vi "QR Code_Read QR Code Setting.vi"(8 "error in":errorcluster, 11 "Buffer Data In":T9) -> (0 "error out":errorcluster, 2 "QR Code Setting":T1={"QR Search Options"={"Rotation Mode"=enum."Unlimited", "Skip Location?"=FALSE, "Edge Threshold"=30, "Demodulation Mode"=-2, "Cell Sample Size"=-2, "Cell Filter Mode"=-2, "Skew Degrees Allowed"=5}, "QR Description Options"={"Matrix Size (cells)"=0, "Barcode Polarity"=-2, "Mirror Mode"=-2, "QR Model"=0}, "QR Code Cell Size (pixels)"={"Minimum Size"=3, "Maximum Size"=7}} {"QR Description Options"."Mirror Mode" items=["Auto-detect"=-2, "Normal"=0, "Mirrored"=1]; "QR Description Options"."Matrix Size (cells)" items=["Auto-detect"=0, "11x11 - Version 1 (Micro QR Only)"=11, "13x13 - Version 2 (Micro QR Only)"=13, "15x15 - Version 3 (Micro QR Only)"=15, "17x17 - Version 4 (Micro QR Only)"=17, "21x21 - Version 1"=21, "25x25 - Version 2"=25, "29x29 - Version 3"=29, "33x33 - Version 4"=33, "37x37 - Version 5"=37, "41x41 - Version 6"=41, "45x45 - Version 7"=45, "49x49 - Version 8"=49, "53x53 - Version 9"=53, "57x57 - Version 10"=57, "61x61 - Version 11"=61, "65x65 - Version 12"=65, "69x69 - Version 13"=69, "73x73 - Version 14"=73, "77x77 - Version 15"=77, "81x81 - Version 16"=81, "85x85 - Version 17"=85, "89x89 - Version 18"=89, "93x93 - Version 19"=93, "97x97 - Version 20"=97, "101x101 - Version 21"=101, "105x105 - Version 22"=105, "109x109 - Version 23"=109, "113x113 - Version 24"=113, "117x117 - Version 25"=117, "121x121 - Version 26"=121, "125x125 - Version 27"=125, "129x129 - Version 28"=129, "133x133 - Version 29"=133, "137x137 - Version 30"=137, "141x141 - Version 31"=141, "145x145 - Version 32"=145, "149x149 - Version 33"=149, "153x153 - Version 34"=153, "157x157 - Version 35"=157, "161x161 - Version 36"=161, "165x165 - Version 37"=165, "169x169 -  Version 38"=169, "173x173 - Version 39"=173, "177x177 - Version 40"=177]; "QR Description Options"."QR Model" items=["Auto-detect", "Micro", "Model 1", "Model 2"]; "QR Description Options"."Barcode Polarity" items=["Auto-detect"=-2, "Black on White"=0, "White on Black"=1]; "QR Search Options"."Cell Filter Mode" items=["Auto-detect"=-2, "Average"=0, "Median"=1, "Central Average"=2, "High Average"=3, "Low Average"=4, "Very High Average"=5, "Very Low Average"=6, "All Filters"=8]; "QR Search Options"."Cell Sample Size" items=["Auto-detect"=-2, "1x1"=1, "2x2"=2, "3x3"=3, "4x4"=4, "5x5"=5, "6x6"=6, "7x7"=7]; "QR Search Options"."Demodulation Mode" items=["Auto-detect"=-2, "Histogram"=0, "Local Contrast"=1, "Combination"=2, "All"=3]}, 3 "Buffer Data Out":T9)   [LabVIEW 2016]
uses:
  Data Def/QR Code_Buffer Data.ctl
  <vilib>/vision/Image Controls.llb/IMAQ Image.ctl
  Data Def/QR Code_QR Code Setting.ctl
  <vilib>/vision/Instrument.llb/QR Code Search Options.ctl
  <vilib>/vision/Instrument.llb/Demodulation Mode.ctl
  <vilib>/vision/Instrument.llb/Cell Sample Size.ctl
  <vilib>/vision/Instrument.llb/Cell Filter Mode.ctl
  <vilib>/vision/Instrument.llb/QR Code Description Options.ctl
  <vilib>/vision/Instrument.llb/Data Matrix Polarity.ctl
  <vilib>/vision/Instrument.llb/QR Code Model Type.ctl
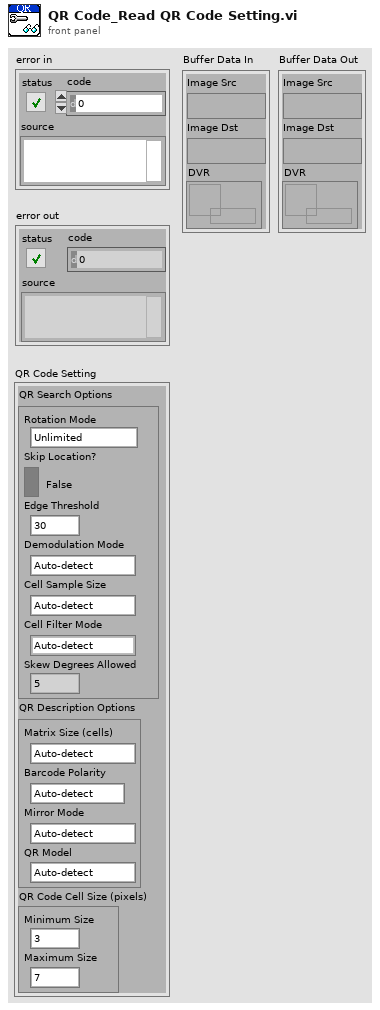
[diagram p1: front panel]
types:
  T1 = typedef "QR Code_QR Code Setting.ctl" = cluster{"QR Search Options":T2, "QR Description Options":T6, "QR Code Cell Size (pixels)":cluster{"Minimum Size":u32, "Maximum Size":u32}}
  T2 = typedef "QR Code Search Options.ctl" = cluster{"Rotation Mode":enum32{"Unlimited", "0 Degrees", "90 Degrees", "180 Degrees", "270 Degrees"}, "Skip Location?":bool, "Edge Threshold":u32, "Demodulation Mode":T3, "Cell Sample Size":T4, "Cell Filter Mode":T5, "Skew Degrees Allowed":u32}
  T3 = typedef "Demodulation Mode.ctl" = i32
  T4 = typedef "Cell Sample Size.ctl" = i32
  T5 = typedef "Cell Filter Mode.ctl" = i32
  T6 = typedef "QR Code Description Options.ctl" = cluster{"Matrix Size (cells)":i32, "Barcode Polarity":T7, "Mirror Mode":i32, "QR Model":T8}
  T7 = typedef "Data Matrix Polarity.ctl" = i32
  T8 = typedef "QR Code Model Type.ctl" = i32
  T9 = typedef "QR Code_Buffer Data.ctl" = cluster{"Image Src":T10, "Image Dst":T10, "DVR":refnum<data-value>}
  T10 = typedef "IMAQ Image.ctl" = refnum<image>
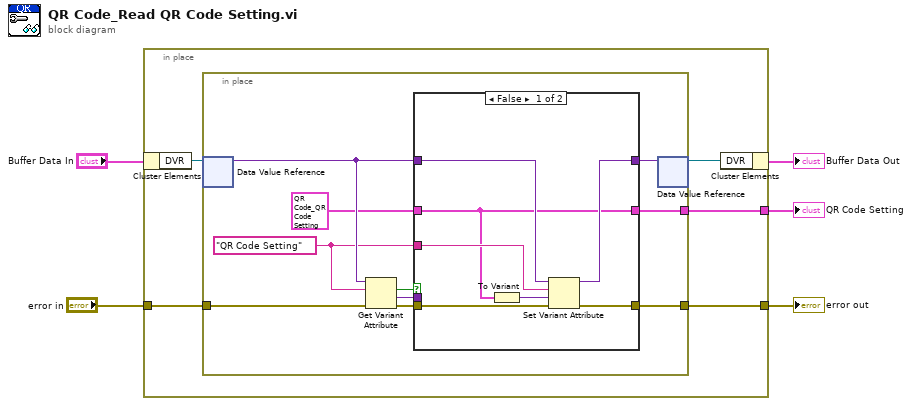
[diagram p0: block diagram]
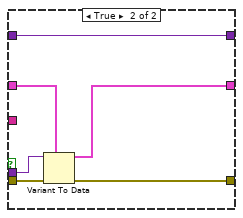
[diagram p2: hidden frame]
diagram:
  n1 = in-place {
    in-place-border: "error in" -> [w9]
    in-place-border: [w7] -> w2
    in-place-border: [w6] -> w1
    n2 = in-place-cluster #1("Buffer Data In") -> ("DVR"=w10:refnum<data-value>)
    n3 = in-place {
      in-place-border: w9 -> [w20]
      in-place-border: [w12] -> w7
      in-place-border: [w11] -> w6
      w15 = "QR Code Setting" ("name")
      n4 = in-place-dvr #2(w10) -> (w16:variant)  [unwired: 1 out]
      n5 = Get Variant Attribute(Variant=w16, name=w15, error in=w20) -> (found=w19:bool, value=w18:variant, error out=w17:errorcluster)  [unwired: 1 in, 1 out]
      n6 = case shown="False" w19 {
        tunnel: w18 -> [_ w31]
        tunnel: w17 -> [w27 w32]
        tunnel: w16 -> [w24 w33]
        tunnel: [w21 w29] -> w11
        tunnel: w15 -> [w25 _]
        tunnel: [w23 w33] -> w14
        tunnel: [w22 w28] -> w12
        tunnel: T1 {"QR Search Options"={"Rotation Mode"=enum."Unlimited", "Skip Location?"=FALSE, "Edge Threshold"=30, "Demodulation Mode"=-2, "Cell Sample Size"=-2, "Cell Filter Mode"=-2, "Skew Degrees Allowed"=5}, "QR Description Options"={"Matrix Size (cells)"=0, "Barcode Polarity"=-2, "Mirror Mode"=-2, "QR Model"=0}, "QR Code Cell Size (pixels)"={"Minimum Size"=3, "Maximum Size"=7}} ("QR Code Setting") -> [w21 w30]
        frame False {
          n7 = To Variant(anything=w21) -> (Variant=w26:variant)
          n8 = Set Variant Attribute(Variant=w24, name=w25, value=w26, error in=w27) -> (Variant out=w23:variant, error out=w22:errorcluster)  [unwired: 1 out]
        }
        frame True {
          n9 = Variant To Data(error in=w32, type=w30, Variant=w31) -> (data=w29:T1, error out=w28:errorcluster)
        }
      }
      n10 = in-place-dvr #2(w14) -> (w8:refnum<data-value>)  [unwired: 1 out]
    }
    n11 = in-place-cluster #1("DVR"=w8) -> (→"Buffer Data Out":T9)
  }
  "error out" <- w2
  "QR Code Setting" <- w1
